vi "Read Ref Value.vi"(8 "error in (no error)":errorcluster, 11 "BetterListboxHandle in":refnum<class "BetterListboxHandle.lvclass">) -> (0 "error out":errorcluster, 2 "Value":i32[](array[numeric]), 3 "BetterListboxHandle out":refnum<class "BetterListboxHandle.lvclass">)   [LabVIEW 2020, in "BetterDragAndDrop.lvlib" / "BetterListboxHandle.lvclass"]
uses:
  BetterListboxHandle.lvclass
  BetterListboxHandle.lvclass/BetterListboxHandle.ctl
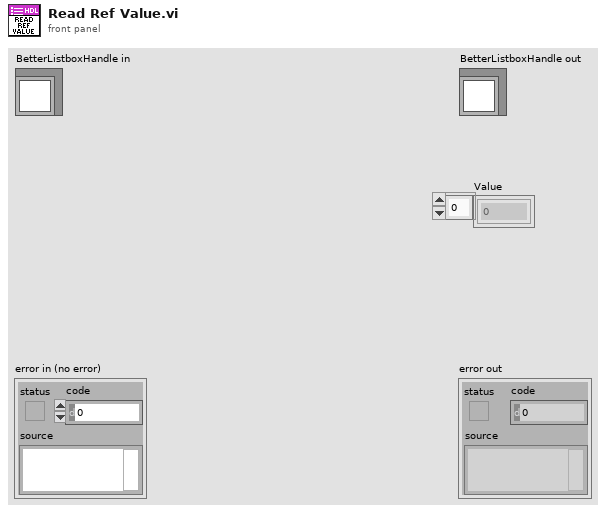
[diagram p1: front panel]
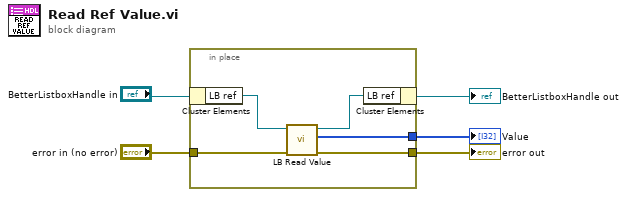
[diagram p0: block diagram]
diagram:
  n1 = in-place {
    in-place-border: "error in (no error)" -> [w9]
    in-place-border: [w8] -> w3
    in-place-border: [w6] -> w1
    n2 = in-place-cluster #1("BetterListboxHandle in") -> ("LB ref"=w10:refnum<vi>)
    n3 = call "LB Read Value.vi"("error in (no error)"=w9, "LB ref (generic)"=w10) -> ("error out"=w8:errorcluster, "Value"=w6:i32[], "LB ref (generic)"=w7:refnum<vi>)  [unwired: 7 in]
    n4 = in-place-cluster #1("LB ref"=w7) -> (→"BetterListboxHandle out":refnum<class "BetterListboxHandle.lvclass">)
  }
  "error out" <- w3
  "Value" <- w1
